vi "Raster_Scan_FSRS.vi"() -> ()   [LabVIEW 2014] (continued)
      n49 = property on="Callibration" class="Bool"("DisabledEnum"=T3."Enabled" ("Disabled")) -> ()  [unwired: 2 in, 2 out]
    }
    frame #2 {
      n50 = while {
        tunnel: w119 -> [w127]
        tunnel: w118 -> [w126]
        tunnel: w117 -> [w125]
        tunnel: w116 -> [w124]
        tunnel: w115 -> [w123]
        tunnel: w114 -> [w122]
        tunnel: w113 -> [w121]
        stop <- "stop" stop-if-true
        n51 = stacked-sequence {
          tunnel: w127 -> [w133 _ _ w229 _ _ _ _]
          tunnel: w126 -> [w132 _ _ w228 _ _ _ _]
          tunnel: w125 -> [w130 _ _ w227 _ _ _ _]
          tunnel: w124 -> [w131 _ _ w226 _ _ _ _]
          tunnel: w123 -> [_ _ _ w223 w358 _ _ _]
          tunnel: w122 -> [w129 _ _ w222 w357 _ _ _]
          tunnel: w121 -> [w128 _ _ w221 w356 _ _ _]
          frame #0 {
            n52 = case shown="True" "winspec" {
              tunnel: w133 -> [_ w142]
              tunnel: w132 -> [_ w141]
              tunnel: w131 -> [_ w139]
              tunnel: w130 -> [_ w138]
              tunnel: w129 -> [_ w136]
              tunnel: w128 -> [_ w135]
              frame False {
              }
              frame True {
                n53 = while {
                  tunnel: w142 -> [w147]
                  tunnel: w141 -> [w148]
                  tunnel: w139 -> [w156]
                  tunnel: w138 -> [w149]
                  stop <- w163 continue-if-true
                  n54 = stacked-sequence {
                    frame #0 {
                      # "This loop continuously updates the graph on the front with the image from the PIXIS"
                      n55 = local read "Camera Handle"() -> (w178:u32)
                      n56 = local read "# Images"() -> (w174:u16)
                      n57 = local read "error out"() -> (w177:errorcluster)
                      n58 = local read "Change to Raman Shift"() -> (w168:bool)
                      n59 = call "DataGrabber.vi"("# Images In"=w174, "Camera Handle"=w178, "error in (no error)"=w177) -> ("# Images Out"=w169:u16, "Camera Handle"=w176:u32, "Data"=w173:dbl[][], "error out"=w175:errorcluster)
                      n60 = case shown="True" w168 {
                        tunnel: [w180 w182] -> w166
                        tunnel: ["Pixel" ("X Scale.Name Label.Text") "Raman Shift (cm-1)" ("X Scale.Name Label.Text")] -> w164
                        frame False {
                          n61 = local read "Result"() -> (w180:dbl[])
                        }
                        frame True {
                          n62 = local read "Result 2"() -> (w182:dbl[])
                        }
                      }
                      n63 = Initialize Array(0.0, u32 1340) -> (w170:dbl[])
                      n64 = call "DataProcessor.vi"("PumpOffBkgd"=w170, "PumpOnBkgd"=w170, "Data"=w173, "# of Images"=w169) -> ("PumpOff"=w167:dbl[])  [unwired: 2 out]
                      n65 = local write "# Images"(w169) -> ()
                      n66 = Build Cluster Array(w166, w167) -> (w165:cluster{dbl, dbl}[])
                      n67 = property on="Spectra" class="XYGraph (strict)"("XScale.NameLbl.Text"=w164) -> ()  [unwired: 2 in, 2 out]
                      n68 = local write "Spectra"(w165) -> ()
                      n69 = local write "Camera Handle"(w176) -> ()
                      n70 = local write "error out"(w175) -> ()
                    }
                    frame #1 {
                      n71 = stacked-sequence {
                        frame #0 {
                          # "Select Cursor 0"
                          n72 = property on="Spectra" class="XYGraph (strict)"("Active Cursor"=0) -> ()  [unwired: 2 in, 2 out]
                        }
                        frame #1 {
                          # "Record the Y position of cursor 0"
                        }
                        frame #2 {
                          # "Select Cursor 1"
                          n73 = property on="Spectra" class="XYGraph (strict)"("Active Cursor"=1) -> ()  [unwired: 2 in, 2 out]
                        }
                        frame #3 {
                          # "Calculate the Gain"
                          n74 = property on="Spectra" class="XYGraph (strict)"() -> ("Cursor.Cursor Position:Cursor Y"=w190:dbl)  [unwired: 2 in, 2 out]
                          n75 = local read "cursor y 2"() -> (w189:dbl)
                          n76 = Subtract(x=w190, y=w189) -> (x-y=w186:dbl)
                          n77 = Absolute Value(x=w186) -> (abs(x)=w188:dbl)
                          n78 = Multiply(x=w188, y=1) -> (x*y=w185:dbl)
                          n79 = local write "Gain"(w185) -> ()
                        }
                      }
                    }
                  }
                  n80 = local read "winspec"() -> (w163:bool)
                  n81 = Boolean To (0,1)(Boolean="PUMP") -> (0, 1=w161:i16)
                  n82 = Multiply(x="Step Size (micro meter)", y=10.0) -> (x*y=w144:dbl)
                  n83 = Add(x=w161, y=i16 1) -> (x+y=w150:i16)
                  n84 = Round To Nearest(number=w144) -> (nearest integer value=w143:dbl)
                  n85 = And(x="MOVE", y=w163) -> (x .and. y?=w157:bool)
                  n86 = call "Pico_move_new.vi"("Motor"=w150, "CmdLib Out"=w147, "DeviceKey Out"=w148, "Start Position"="Start Position", "Boolean 2"="GO", "Relative Steps"=w143, "Boolean"=w157, "error out"=w156, "Device Address Out"=w149) -> ("CmdLib Out"=→"CmdLib Out":refnum<k24>, "DeviceKey Out"=→"DeviceKey Out":string, "Device Address Out"=→"Device Address Out":i32, "error out 2"=→"error out 2":errorcluster)  [unwired: 3 in]
                }
                n87 = call "shutter_new.vi"("error in"=w135, "ShutterID"=310, "Shutter Position"="Shutter Position", "ObjectPtr"=w136) -> ()  [unwired: 1 out]
              }
            }
          }
          frame #1 {
            n88 = case shown="True" "Bkgnd" {
              frame False {
              }
              frame True {
                # "Process the Data"
                # "Get the data!"
                # "Display the Raman Pump on graph on the Front Panel and store data"
                n89 = local read "Camera Handle"() -> (w205:u32)
                n90 = local read "# Images"() -> (w200:u16)
                n91 = local read "error out"() -> (w204:errorcluster)
                n92 = local read "Change to Raman Shift"() -> (w193:bool)
                n93 = call "DataGrabber.vi"("# Images In"=w200, "Camera Handle"=w205, "error in (no error)"=w204) -> ("# Images Out"=w197:u16, "Camera Handle"=w203:u32, "Data"=w201:dbl[][], "error out"=w202:errorcluster)
                n94 = local write "Camera Handle"(w203) -> ()
                n95 = local write "error out"(w202) -> ()
                n96 = local write "# Images"(w197) -> ()
                n97 = case shown="True" w193 {
                  tunnel: [w209 w211] -> w196
                  tunnel: ["Pixel" ("X Scale.Name Label.Text") "Raman Shift (cm-1)" ("X Scale.Name Label.Text")] -> w192
                  frame False {
                    n98 = local read "Result"() -> (w209:dbl[])
                  }
                  frame True {
                    n99 = local read "Result 2"() -> (w211:dbl[])
                  }
                }
                n100 = Initialize Array(0.0) -> (w198:dbl[])  [unwired: 1 in]
                n101 = call "DataProcessor.vi"("PumpOffBkgd"=w198, "PumpOnBkgd"=w198, "Data"=w201, "# of Images"=w197) -> ("PumpOff"=→"Bkgndoff":dbl[], "PumpOn"=→"Bkgndon":dbl[], "Raman"=w195:dbl[])
                n102 = Build Cluster Array(w196, w195) -> (w194:cluster{dbl, dbl}[])
                n103 = property on="Spectra" class="XYGraph (strict)"("XScale.NameLbl.Text"=w192) -> ()  [unwired: 2 in, 2 out]
                n104 = local write "Spectra"(w194) -> ()
              }
            }
          }
          frame #2 {
            n105 = case shown="True" "Callibration" {
              frame False {
              }
              frame True {
                n106 = for {
                  N: 1340 -> [_]
                  tunnel: [w220] -> w219 mode=indexing
                  i -> [w220]
                }
                n107 = call "cal.vi"("array"=w219, "Laser Wavelength"="Laser Wavelength (nm)", "Wave Number"="Shift", "Pixel"="Pixel") -> ("array 2"=→"Result":dbl[], "Result"=→"Result 2":dbl[])  [unwired: 6 in]
              }
            }
          }
          frame #3 {
            n108 = Compound Arithmetic op=OR("Acquire", "Focus") -> (w230:bool)
            n109 = case shown="True" w230 {
              selector: w230 -> [_ w238]
              tunnel: w229 -> [_ w237]
              tunnel: w228 -> [_ w236]
              tunnel: w227 -> [_ w235]
              tunnel: w226 -> [_ w234]
              tunnel: w223 -> [_ w233]
              tunnel: w222 -> [_ w232]
              tunnel: w221 -> [_ w231]
              frame False {
              }
              frame True {
                n110 = while {
                  tunnel: w238 -> [w276]
                  tunnel: w237 -> [w268]
                  tunnel: w236 -> [w267]
                  tunnel: w235 -> [w266]
                  tunnel: w234 -> [w265]
                  tunnel: w233 -> [w244]
                  tunnel: w232 -> [w240]
                  tunnel: w231 -> [w239]
                  stop <- w243 continue-if-true
                  n111 = stacked-sequence {
                    seq-local: [w288 _ _ _] -> [_ w311 _ _]
                    seq-local: [w293 _ _ _] -> [_ w308 _ _]
                    frame #0 {
                      n112 = local read "Camera Handle"() -> (w297:u32)
                      n113 = local read "# Images"() -> (w298:u16)
                      n114 = local read "error out"() -> (w296:errorcluster)
                      n115 = local read "Change to Raman Shift"() -> (w284:bool)
                      n116 = call "DataGrabber.vi"("# Images In"=w298, "Camera Handle"=w297, "error in (no error)"=w296) -> ("# Images Out"=w288:u16, "Camera Handle"=w294:u32, "Data"=w293:dbl[][], "error out"=w295:errorcluster)
                      n117 = case shown="False" w284 {
                        tunnel: [w300 w302] -> w282
                        tunnel: ["Pixel" ("X Scale.Name Label.Text") "Raman Shift (cm-1)" ("X Scale.Name Label.Text")] -> w285
                        frame False {
                          n118 = local read "Result"() -> (w300:dbl[])
                        }
                        frame True {
                          n119 = local read "Result 2"() -> (w302:dbl[])
                        }
                      }
                      n120 = local write "Camera Handle"(w294) -> ()
                      n121 = local write "error out"(w295) -> ()
                      n122 = Initialize Array(0.0, u32 1340) -> (w290:dbl[])
                      n123 = call "DataProcessor.vi"("PumpOffBkgd"=w290, "PumpOnBkgd"=w290, "Data"=w293, "# of Images"=w288) -> ("PumpOff"=w280:dbl[], "PumpOn"=w289:dbl[], "Raman"=w286:dbl[])
                      n124 = local write "# Images"(w288) -> ()
                      n125 = local write "Waveform Graph"(w280) -> ()
                      n126 = property on="Spectra" class="XYGraph (strict)"("XScale.NameLbl.Text"=w285) -> ()  [unwired: 2 in, 2 out]
                      n127 = local write "On"(w289) -> ()
                      n128 = local write "Off"(w280) -> ()
                      n129 = case shown="True" "Flip Spectra" {
                        tunnel: [w303 w304] -> w283
                        tunnel: w286 -> [w303 w305]
                        frame False {
                        }
                        frame True {
                          # "Flip Displayed Spectra"
                          n130 = Reciprocal(x=w305) -> (1/x=w304:dbl[])
                        }
                      }
                      n131 = local write "Raman"(w286) -> ()
                      n132 = Build Cluster Array(w282, w283) -> (w281:cluster{dbl, dbl}[])
                      n133 = local write "Spectra"(w281) -> ()
                    }
                    frame #1 {
                      w315 = 2
                      n134 = Initialize Array(0.0, u32 1340) -> (w319:dbl[])
                      n135 = Initialize Array(0.0, u32 1340) -> (w320:dbl[])
                      n136 = Subtract(x=w311, y=u16 10) -> (x-y=w310:u16)
                      n137 = Divide(x=w311, y=w315) -> (x/y=w316:dbl)
                      n138 = Delete From Array(array=w308, length=10, index (row)=0) -> (array with subset deleted=w307:dbl[][])  [unwired: 1 in, 1 out]
                      n139 = for {
                        N: w310 -> [_]
                        tunnel: w307 -> [w331]
                        shift-right: [w329] -> w318
                        shift-left: w320 -> [w330]
                        shift-right: [w327] -> w317
                        shift-left: w319 -> [w328]
                        tunnel: w315 -> [w326]
                        i -> [w325]
                        n140 = Quotient & Remainder(x=w325, y=w326) -> (x-y*floor(x/y)=w333:i32)  [unwired: 1 out]
                        n141 = Equal To 0?(x=w333) -> (x = 0?=w332:bool)
                        n142 = case shown="True" w332 {
                          tunnel: w331 -> [w338 w345]
                          tunnel: w330 -> [w339 w343]
                          tunnel: [w339 w342] -> w329
                          tunnel: w328 -> [w337 w341]
                          tunnel: [w335 w341] -> w327
                          tunnel: w325 -> [w334 w340]
                          frame False {
                            # "Raman Pump Off\nOdd Images"
                            n143 = Index Array(array=w338, index (row)=w334) -> (element=w336:dbl[])  [unwired: 1 in]
                            n144 = Add(x=w336, y=w337) -> (x+y=w335:dbl[])
                          }
                          frame True {
                            # "Raman pump on\nEven Images"
                            n145 = Index Array(array=w345, index (row)=w340) -> (element=w344:dbl[])  [unwired: 1 in]
                            n146 = Add(x=w344, y=w343) -> (x+y=w342:dbl[])
                          }
                        }
                      }
                      n147 = Divide(x=w318, y=w316) -> (x/y=w313:dbl[])
                      n148 = Divide(x=w317, y=w316) -> (x/y=w314:dbl[])
                      n149 = Divide(x=w313, y=w314) -> ()  [unwired: 1 out]
                    }
                    frame #2 {
                      # "Calculate the Gain based on the two cursors on the graph"
                      n150 = stacked-sequence {
                        frame #0 {
                          # "Select Cursor 0"
                          n151 = property on="Spectra" class="XYGraph (strict)"("Active Cursor"=0) -> ()  [unwired: 2 in, 2 out]
                        }
                        frame #1 {
                          # "Record the Y position of cursor 0"
                          n152 = property on="Spectra" class="XYGraph (strict)"() -> ("Cursor.Cursor Position:Cursor Y"=→"cursor y":dbl)  [unwired: 2 in, 2 out]
                        }
                        frame #2 {
                          # "Select Cursor 1"
                          n153 = property on="Spectra" class="XYGraph (strict)"("Active Cursor"=1) -> ()  [unwired: 2 in, 2 out]
                        }
                        frame #3 {
                          # "Calculate the Gain"
                          n154 = property on="Spectra" class="XYGraph (strict)"() -> ("Cursor.Cursor Position:Cursor Y"=w349:dbl)  [unwired: 2 in, 2 out]
                          n155 = local read "cursor y"() -> (w354:dbl)
                          n156 = Subtract(x=w349, y=w354) -> (x-y=w351:dbl)
                          n157 = Absolute Value(x=w351) -> (abs(x)=w353:dbl)
                          n158 = Multiply(x=w353, y=100) -> (x*y=→"Gain":dbl)
                        }
                      }
                    }
                    frame #3 {
                      n159 = Wait (ms)(milliseconds to wait=50) -> ()  [unwired: 1 out]
                    }
                  }
                  n160 = call <instrlib>:"_subvi_LivePos_Main.vi"("xCommand"="xCommand", "yCommand"="yCommand", "zCommand"="zCommand", "handle"=w244, "commandZ"="commandZ", "commandY"="commandY", "commandX"="commandX") -> ("xRead"=w255:dbl, "yRead"=w254:dbl, "zRead"=w253:dbl, "counter"=w245:u32)  [unwired: 1 in, 8 out]
                  n161 = Equal To 0?(x=w245) -> (x = 0?=w246:bool)
                  n162 = case shown="True" w246 {
                    tunnel: w255 -> [_ w279]
                    tunnel: w254 -> [_ w278]
                    tunnel: w253 -> [_ w277]
                    frame False {
                    }
                    frame True {
                      "xRead" <- w279
                      "yRead" <- w278
                      "zRead" <- w277
                    }
                  }
                  n163 = local read "Shutter Position"() -> (w242:bool)
                  n164 = local read "Focus"() -> (w243:bool)
                  n165 = local read "Step Size (micro meter)"() -> (w259:dbl)
                  n166 = local read "Start Position"() -> (w270:i32)
                  n167 = local read "MOVE"() -> (w272:bool)
                  n168 = local read "PUMP"() -> (w273:bool)
                  n169 = local read "GO"() -> (w264:bool)
                  n170 = Boolean To (0,1)(Boolean=w273) -> (0, 1=w275:i16)
                  n171 = call "shutter_new.vi"("error in"=w239, "ShutterID"=310, "Shutter Position"=w242, "ObjectPtr"=w240) -> ()  [unwired: 1 out]
                  n172 = Add(x=w275, y=i16 1) -> (x+y=w271:i16)
                  n173 = And(x=w272, y=w276) -> (x .and. y?=w269:bool)
                  n174 = Multiply(x=w259, y=10.0) -> (x*y=w257:dbl)
                  n175 = Round To Nearest(number=w257) -> (nearest integer value=w256:dbl)
                  n176 = call "Pico_move_new.vi"("Motor"=w271, "CmdLib Out"=w268, "DeviceKey Out"=w267, "Start Position"=w270, "Boolean 2"=w264, "Relative Steps"=w256, "Boolean"=w269, "error out"=w265, "Device Address Out"=w266) -> ("CmdLib Out"=w263:refnum<k24>, "DeviceKey Out"=w262:string, "Device Address Out"=w261:i32, "error out 2"=w260:errorcluster)  [unwired: 3 in]
                  n177 = local write "CmdLib Out"(w263) -> ()
                  n178 = local write "Device Address Out"(w261) -> ()
                  n179 = local write "error out 2"(w260) -> ()
                  n180 = local write "DeviceKey Out"(w262) -> ()
                }
              }
            }
          }
          frame #4 {
            n181 = case shown="True" "Ruster Scan" {
              tunnel: w358 -> [_ w402]
              tunnel: w357 -> [_ w376]
              tunnel: w356 -> [_ w375]
              frame False {
                (unwired) FALSE ("Pause 2")
              }
              frame True {
                w394 = dbl[][] []
                # "X Ramp Generator"
                # "Y Ramp Generator"
                n182 = local read "Path"() -> (w362:string)
                n183 = Build Array("X Start  (um)", "X End  (um)", "Y Start  (um)", "Y End  (um)") -> (w393:dbl[])
                n184 = Concatenate Strings(w362, "\\" ("string"), "OFF" ("string")) -> (w364:string)
                n185 = Concatenate Strings("Path", "\\" ("string"), "ON" ("string")) -> (w369:string)
                n186 = Array Max & Min(array=w393) -> (max value=w387:dbl)  [unwired: 3 out]
                n187 = String To Path(string=w364) -> (path=w367:path)
                n188 = String To Path(string=w369) -> (path=w373:path)
                n189 = call "RampGenerator.vi"("Number of Positions"="Y Samples", "End  (um)"="Y End  (um)", "Start  (um)"="Y Start  (um)") -> ("Array"=w396:dbl[])  [unwired: 1 in]
                n190 = Greater?(x=w387, y=70.0) -> (0:w377:bool)
                n191 = call "RampGenerator.vi"("Number of Positions"="X Samples", "End  (um)"="X End  (um)", "Start  (um)"="X Start  (um)") -> ("Array"=w397:dbl[])  [unwired: 1 in]
                n192 = case shown="True" w377 {
                  tunnel: [w404 w406] -> w398
                  tunnel: w396 -> [w404 _]
                  tunnel: [w403 w406] -> w399
                  tunnel: w397 -> [w403 _]
                  frame False {
                  }
                  frame True {
                    w406 = dbl[] [] ("Array")
                    n193 = One Button Dialog(message="Values are \nout of Range") -> ()  [unwired: 1 in, 1 out]
                  }
                }
                n194 = Create Folder(path (use dialog)=w367) -> (created path=w363:path)  [unwired: 2 in, 2 out]
                n195 = Create Folder(path (use dialog)=w373) -> (created path=w368:path)  [unwired: 2 in, 2 out]
                n196 = Path To String(path=w363) -> (string=→"OFF":string)
                n197 = Path To String(path=w368) -> (string=→"ON":string)
                n198 = Array Size(array=w396) -> (size(s)=w395:i32)
                n199 = while {
                  tunnel: w398 -> [w448]
                  tunnel: w402 -> [w447]
                  tunnel: w399 -> [w446]
                  tunnel: "X Start  (um)" -> [w445]
                  shift-right: [w440] -> w378
                  shift-left: w394 -> [w424]
                  shift-right: [w442] -> w382
                  shift-left: w394 -> [w423]
                  tunnel: w377 -> [w414]
                  tunnel: w395 -> [w438]
                  tunnel: "X Start  (um)" -> [w437]
                  tunnel: "X End  (um)" -> [w436]
                  tunnel: "Y Start  (um)" -> [w435]
                  tunnel: "Y End  (um)" -> [w434]
                  shift-right: [w429] -> w383
                  shift-left: w394 -> [w425]
                  shift-right: [w427] -> w386
                  shift-left: w394 -> [w426]
                  tunnel: w376 -> [w412]
                  tunnel: w375 -> [w411]
                  i -> [w444]
                  stop <- w413 stop-if-true
                  n200 = Bundle(w426, w425, w424, w423, w414) -> (w422:T5)  [unwired: 1 in]
                  n201 = Unbundle(w422) -> (w421:dbl[][], w418:dbl[][], w420:dbl[][], w419:dbl[][], w410:bool)
                  n202 = stacked-sequence {
                    seq-local: [w450 _] -> [_ w477]
                    tunnel: w448 -> [w454 _]
                    tunnel: w444 -> [w452 w464]
                    tunnel: w447 -> [w453 w478]
                    tunnel: w446 -> [_ w480]
                    tunnel: w445 -> [_ w479]
                    tunnel: [w451 _] -> w408
                    tunnel: [_ w476] -> w417
                    tunnel: [_ w475] -> w416
                    tunnel: [_ w463] -> w433
                    tunnel: w414 -> [_ w474]
                    tunnel: w410 -> [_ w473]
                    tunnel: w438 -> [_ w472]
                    tunnel: w437 -> [_ w471]
                    tunnel: w436 -> [_ w470]
                    tunnel: w435 -> [_ w469]
                    tunnel: w434 -> [_ w468]
                    tunnel: [_ w466] -> w415
                    tunnel: [_ w465] -> w432
                    tunnel: w412 -> [_ w462]
                    tunnel: w411 -> [_ w461]
                    tunnel: [_ w460] -> w407
                    frame #0 {
                      w457 = 2  # Y AXIS
                      # "Step the Y axis"
                      n203 = Array Size(array=w454) -> (size(s)=w449:i32)
                      n204 = Index Array(array=w454, index=w452) -> (element=w455:dbl)
                      n205 = Increment(x=w452) -> (x+1=w456:i32)
                      n206 = Subtract(x=w449, y=w456) -> (x-y=w459:i32)
                      n207 = Equal To 0?(x=w459) -> (x = 0?=w451:bool)
                      n208 = call "WriteReadN.vi"("Handle"=w453, "Axis"=w457, "Delay (ms)"="Y Delay (ms)", "Move to (um)"=w455) -> ("Current Position (um)"=w450:dbl)
                      "Y Position (um)" <- w450
                    }
                    frame #1 {
                      w467 = dbl[] []
                      n209 = while {
                        tunnel: w480 -> [w514]
                        tunnel: w479 -> [w513]
                        tunnel: w478 -> [w511]
                        tunnel: w477 -> [w510]
                        tunnel: w464 -> [w497]
                        shift-right: [w509] -> w476
                        shift-left: w467 -> [w496]
                        shift-right: [w508] -> w475
                        shift-left: w467 -> [w495]
                        tunnel: w474 -> [w507]
                        tunnel: w473 -> [w505]
                        tunnel: w472 -> [w504]
                        tunnel: w471 -> [w503]
                        tunnel: w470 -> [w502]
                        tunnel: w469 -> [w501]
                        tunnel: w468 -> [w500]
                        shift-right: [w499] -> w466
                        shift-left: w467 -> [w494]
                        shift-right: [w498] -> w465
                        shift-left: w467 -> [w490]
                        tunnel: w464 -> [w487]
                        tunnel: [w486] -> w463
                        tunnel: w462 -> [w485]
                        tunnel: w461 -> [w484]
                        tunnel: [w481] -> w460
                        i -> [w512]
                        stop <- w506 stop-if-true
                        n210 = Bundle(w496, w495, w490, w494, w487) -> (w493:cluster{dbl[], dbl[], dbl[], dbl[], i32})  [unwired: 1 in]
                        n211 = Unbundle(w493) -> (w492:dbl[], w491:dbl[], w489:dbl[], w488:dbl[], w486:i32)
                        n212 = stacked-sequence {
                          seq-local: [w532 _] -> [_ w572]
                          tunnel: w514 -> [w537 _]
                          tunnel: w513 -> [_ _]
                          tunnel: w512 -> [w528 _]
                          tunnel: w511 -> [w545 _]
                          tunnel: [w544 _] -> w483
                          tunnel: w510 -> [w543 w573]
                          tunnel: w497 -> [w530 _]
                          tunnel: w492 -> [_ w564]
                          tunnel: [_ w563] -> w509
                          tunnel: [_ w557] -> w508
                          tunnel: w491 -> [_ w566]
                          tunnel: w507 -> [_ _]
                          tunnel: w504 -> [w531 _]
                          tunnel: w503 -> [w520 _]
                          tunnel: w502 -> [w519 _]
                          tunnel: w501 -> [w517 _]
                          tunnel: w500 -> [w518 _]
                          tunnel: w488 -> [_ w561]
                          tunnel: [_ w560] -> w499
                          tunnel: w489 -> [_ w569]
                          tunnel: [_ w567] -> w498
                          tunnel: w485 -> [_ w556]
                          tunnel: w484 -> [_ w555]
                          tunnel: [_ w554] -> w481
                          frame #0 {
                            w546 = 1  # X AXIS
                            # "Step the X axis"
                            n213 = Quotient & Remainder(x=w530, y=2) -> (x-y*floor(x/y)=w541:i32)  [unwired: 1 out]
                            n214 = Array Size(array=w537) -> (size(s)=w529:i32)
                            n215 = Equal?(x=w541, y=0) -> (x = y?=w534:bool)
                            n216 = Multiply(x=w529, y=w530) -> (x*y=w526:i32)
                            n217 = Increment(x=w528) -> (x+1=w527:i32)
                            n218 = Subtract(x=w529, y=1) -> (x-y=w535:i32)
                            n219 = Add(x=w526, y=w527) -> (x+y=w523:i32)
                            n220 = Multiply(x=w531, y=w529) -> (x*y=w522:i32)
                            n221 = Divide(x=w523, y=w522) -> (x/y=w525:dbl)
                            n222 = Subtract(x=w535, y=w528) -> (x-y=w538:i32)
                            n223 = case shown="False" w534 {
                              tunnel: w537 -> [w549 w553]
                              tunnel: w528 -> [_ w552]
                              tunnel: [w550 w551] -> w539
                              tunnel: w538 -> [w548 _]
                              frame False {
                                n224 = Index Array(array=w549, index=w548) -> (element=w550:dbl)
                              }
                              frame True {
                                n225 = Index Array(array=w553, index=w552) -> (element=w551:dbl)
                              }
                            }
                            n226 = Multiply(x=w525, y=100.0) -> (x*y=→"Progress (%)":dbl)
                            n227 = Equal To 0?(x=w538) -> (x = 0?=w544:bool)
                            n228 = Not Equal?(x=w522, y=w523) -> (x != y?=w516:bool)
                            "?" <- w516
                            n229 = call "WriteReadN.vi"("Handle"=w545, "Axis"=w546, "Delay (ms)"="X Deyal (ms)", "Move to (um)"=w539) -> ("Current Position (um)"=w532:dbl)
                            "X Position (um)" <- w532
                            n230 = Not(x=w516) -> (.not. x?=w521:bool)
                            n231 = call "?"("Reset"=w521, "Y Input"=w543, "X Input"=w532) -> ("XY Graph"=→"XY Graph":cluster{"X":dbl[], "Y":dbl[]}[])  [unwired: 7 in, 1 out]
                            n232 = property on="XY Graph" class="XYGraph (strict)"("XScale.Maximum"=w519) -> ()  [unwired: 2 in, 2 out]
                            n233 = property on="XY Graph" class="XYGraph (strict)"("YScale.Minimum"=w517) -> ()  [unwired: 2 in, 2 out]
                            n234 = property on="XY Graph" class="XYGraph (strict)"("YScale.Maximum"=w518) -> ()  [unwired: 2 in, 2 out]
                            n235 = property on="XY Graph" class="XYGraph (strict)"("XScale.Minimum"=w520) -> ()  [unwired: 2 in, 2 out]
                          }
                          frame #1 {
                            w570 = 0.0
                            w571 = 0.0
                            n236 = for {
                              N: "Sets" -> [w593]
                              tunnel: w572 -> [w603]
                              tunnel: w573 -> [w602]
                              shift-right: [w600] -> w562
                              shift-left: w571 -> [w588]
                              shift-right: [w599] -> w565
                              shift-left: w570 -> [w587]
                              shift-right: [w595] -> w568
                              shift-left: w571 -> [w589]
                              shift-right: [w594] -> w558
                              shift-left: w570 -> [w590]
                              tunnel: w556 -> [w580]
                              tunnel: w555 -> [w579]
                              tunnel: [w575] -> w554
                              i -> [w604]
                              n237 = Increment(x=w604) -> (x+1=w581:i32)
                              "Current Set" <- w581
                              n238 = local read item#69() -> (w591:bool)
                              n239 = Bundle(w590, w589, w588, w587) -> (w586:cluster{dbl, dbl, dbl, dbl})  [unwired: 1 in]
                              n240 = Not Equal?(x=w593, y=w581) -> (x != y?=w592:bool)
                              n241 = Not Or(1:w591, 2:w592) -> (0:w577:bool)
                              n242 = Not(x=w577) -> (.not. x?=w576:bool)
                              n243 = stacked-sequence {
                                tunnel: w581 -> [w605 _ _]
                                tunnel: w603 -> [w613 _ _]
                                tunnel: w602 -> [w612 _ _]
                                tunnel: [w611 _ _] -> w601
                                tunnel: [w610 _ _] -> w598
                                tunnel: [w609 _ _] -> w597
                                tunnel: [w608 _ _] -> w596
                                tunnel: w580 -> [w607 _ _]
                                tunnel: w579 -> [w606 _ _]
                                tunnel: [_ _ "STOP Scan"] -> w575
                                frame #0 {
                                n244 = stacked-sequence {
                                seq-local: [_ "# Images" _ _ _ _ _ _] -> [_ _ _ _ _ w698 _ _]
                                seq-local: [_ w622 _ _ _ _ _ _] -> [_ _ w650 _ _ _ w719 _]
                                tunnel: w613 -> [_ _ _ w673 _ _ _ w740]
                                tunnel: w612 -> [_ _ _ w672 _ _ _ w739]
                                tunnel: [_ _ w652 _ _ _ _ _] -> w611
                                tunnel: [_ _ w651 _ _ _ _ _] -> w610
                                tunnel: w605 -> [_ _ _ w674 _ _ _ w741]
                                tunnel: [_ _ _ _ _ _ w718 _] -> w609
                                tunnel: [_ _ _ _ _ _ w717 _] -> w608
                                tunnel: w607 -> [w615 _ _ _ w682 _ _ _]
                                tunnel: w606 -> [w614 _ _ _ w681 _ _ _]
                                frame #0 {
                                n245 = flat-sequence {
                                tunnel: w615 -> [w619]
                                tunnel: w614 -> [w618]
                                frame #0 {
                                n246 = call "shutter_new.vi"("error in"=w618, "ShutterID"=310, "Shutter Position"=TRUE, "ObjectPtr"=w619) -> ()  [unwired: 1 out]
                                }
                                frame #1 {
                                n247 = Wait (ms)(milliseconds to wait=u32 200) -> ()  [unwired: 1 out]
                                }
                                }
                                }
                                frame #1 {
                                n248 = local read "Camera Handle"() -> (w639:u32)
                                n249 = local read "error out"() -> (w638:errorcluster)
                                n250 = call "DataGrabber.vi"("# Images In"="# Images", "Camera Handle"=w639, "error in (no error)"=w638) -> ("# Images Out"=w632:u16, "Camera Handle"=w636:u32, "Data"=w635:dbl[][], "error out"=w637:errorcluster)
                                n251 = case shown="True" "Change to Raman Shift" {
                                tunnel: [w641 w643] -> w622
                                tunnel: ["Pixel" ("X Scale.Name Label.Text") "Raman Shift (cm-1)" ("X Scale.Name Label.Text")] -> w625
                                frame False {
                                n252 = local read "Result"() -> (w641:dbl[])
                                }
                                frame True {
                                n253 = local read "Result 2"() -> (w643:dbl[])
                                }
                                }
                                n254 = local write "Camera Handle"(w636) -> ()
                                n255 = local write "error out"(w637) -> ()
                                n256 = local write "# Images"(w632) -> ()
                                n257 = local read "Bkgndoff"() -> (w633:dbl[])
                                n258 = local read "Bkgndon"() -> (w634:dbl[])
                                n259 = call "DataProcessor.vi"("PumpOffBkgd"=w633, "PumpOnBkgd"=w634, "Data"=w635, "# of Images"=w632) -> ("PumpOff"=w621:dbl[], "PumpOn"=w630:dbl[], "Raman"=w629:dbl[])
                                "Ground" <- w629
                                "On" <- w630
                                "Off" <- w621
                                "Raman" <- w629
                                n260 = local read "Flip Spectra"() -> (w624:bool)
                                n261 = local write "Waveform Graph"(w621) -> ()
                                n262 = property on="Spectra" class="XYGraph (strict)"("XScale.NameLbl.Text"=w625) -> ()  [unwired: 2 in, 2 out]
                                n263 = local write "On"(w630) -> ()
                                n264 = local write "Off"(w621) -> ()
                                n265 = Not(x=w624) -> (.not. x?=w623:bool)
                                n266 = case shown="True" w623 {
                                tunnel: w629 -> [w644 w646]
                                tunnel: [w645 w646] -> w628
                                frame False {
                                n267 = Reciprocal(x=w644) -> (1/x=w645:dbl[])
                                }
                                frame True {
                                }
                                }
                                n268 = Build Cluster Array(w622, w628) -> (→"Spectra":cluster{dbl, dbl}[])
                                }
                                frame #2 {
                                # "Peak fitting and intergation"
                                n269 = local read "Raman"() -> (w653:dbl[])
                                n270 = property on="Spectra" class="XYGraph (strict)"("Active Cursor"=u32 1) -> ("Cursor.Cursor X"=w655:dbl)  [unwired: 2 in, 2 out]
                                n271 = property on="Spectra" class="XYGraph (strict)"("Active Cursor"=u32 0) -> ("Cursor.Cursor X"=w656:dbl)  [unwired: 2 in, 2 out]
                                n272 = call "fit_new.vi"("Filter ?"="Filter?", "parameter bounds"="parameter bounds", "Cursor1 2"=w655, "Cursor1"=w656, "array 2"=w650, "array"=w653, "Enum"="Enum", "Initial Parameters"="Initial Parameters") -> ("Intergrate"=w651:dbl, "Fit"=w652:dbl)  [unwired: 2 in]
                                "FIT" <- w652
                                "AREA" <- w651
                                }
                                frame #3 {
                                # "Here we save spectrum for each special point"
                                n273 = local read "ON"() -> (w667:string)
                                n274 = Format Into String(w674) -> (resulting string=w660:string)  [unwired: 3 in, 1 out]
                                n275 = call "number_to_sring.vi"("Numeric"=w673) -> ("result string"=w665:string)  [unwired: 10 in]
                                n276 = call "number_to_sring.vi"("Numeric"=w672) -> ("result string"=w663:string)  [unwired: 10 in]
                                n277 = Concatenate Strings(w667, "\\", "Filename", "_", "X_" ("string"), w665, "_Y_" ("string"), w663, "_ON" ("string"), "_" ("string"), w660) -> (w671:string)
                                "File_name" <- w671
                                n278 = local read "Ground"() -> (w659:dbl[])
                                n279 = local read "On"() -> (w680:dbl[])
                                n280 = local read "Off"() -> (w679:dbl[])
                                n281 = String To Path(string=w671) -> (path=w677:path)
                                n282 = Build Array(w659, w680, w679) -> (w678:dbl[][])
                                n283 = call-poly <vilib>:"Write To Spreadsheet File.vi"("transpose? (no:F)"=TRUE, "format (%.3f)"="%.7f", "2D data"=w678, "file path (dialog if empty)"=w677) -> ()  [unwired: 4 in, 1 out]
                                }
                                frame #4 {
                                n284 = flat-sequence {
                                tunnel: w682 -> [w686]
                                tunnel: w681 -> [w685]
                                frame #0 {
                                n285 = call "shutter_new.vi"("error in"=w685, "ShutterID"=310, "Shutter Position"=FALSE, "ObjectPtr"=w686) -> ()  [unwired: 1 out]
                                }
                                frame #1 {
                                n286 = Wait (ms)(milliseconds to wait=u32 200) -> ()  [unwired: 1 out]
                                }
                                }
                                }
                                frame #5 {
                                n287 = local read "Camera Handle"() -> (w706:u32)
                                n288 = local read "error out"() -> (w705:errorcluster)
                                n289 = local read "Change to Raman Shift"() -> (w694:bool)
                                n290 = call "DataGrabber.vi"("# Images In"=w698, "Camera Handle"=w706, "error in (no error)"=w705) -> ("# Images Out"=w699:u16, "Camera Handle"=w703:u32, "Data"=w702:dbl[][], "error out"=w704:errorcluster)
                                n291 = local write "Camera Handle"(w703) -> ()
                                n292 = local write "error out"(w704) -> ()
                                n293 = local write "# Images"(w699) -> ()
                                n294 = local read "Bkgndoff"() -> (w700:dbl[])
                                n295 = local read "Bkgndon"() -> (w701:dbl[])
                                n296 = case shown="False" w694 {
                                tunnel: [w708 w710] -> w693
                                tunnel: ["Pixel" ("X Scale.Name Label.Text") "Raman Shift (cm-1)" ("X Scale.Name Label.Text")] -> w695
                                frame False {
                                n297 = local read "Result"() -> (w708:dbl[])
                                }
                                frame True {
                                n298 = local read "Result 2"() -> (w710:dbl[])
                                }
                                }
                                n299 = call "DataProcessor.vi"("PumpOffBkgd"=w700, "PumpOnBkgd"=w701, "Data"=w702, "# of Images"=w699) -> ("PumpOff"=w688:dbl[], "PumpOn"=w697:dbl[], "Raman"=w696:dbl[])
                                n300 = local read "Flip Spectra"() -> (w690:bool)
                                n301 = local write "Waveform Graph"(w688) -> ()
                                n302 = Not(x=w690) -> (.not. x?=w689:bool)
                                n303 = local write "On"(w697) -> ()
                                n304 = local write "Off"(w688) -> ()
                                n305 = case shown="True" w689 {
                                tunnel: w696 -> [w712 w713]
                                tunnel: [w711 w713] -> w692
                                frame False {
                                n306 = Reciprocal(x=w712) -> (1/x=w711:dbl[])
                                }
                                frame True {
                                }
                                }
                                n307 = property on="Spectra" class="XYGraph (strict)"("XScale.NameLbl.Text"=w695) -> ()  [unwired: 2 in, 2 out]
                                n308 = local write "Ground"(w696) -> ()
                                n309 = local write "Raman"(w696) -> ()
                                n310 = Build Cluster Array(w693, w692) -> (w691:cluster{dbl, dbl}[])
                                n311 = local write "Off"(w688) -> ()
                                n312 = local write "Spectra"(w691) -> ()
                                n313 = local write "On"(w697) -> ()
                                }
                                frame #6 {
                                # "Peak fitting and intergation"
                                n314 = local read "Raman"() -> (w720:dbl[])
                                n315 = local read "Initial Parameters"() -> (w721:T2)
                                n316 = local read "Enum"() -> (w716:enum16{"Lorantzian", "fano", "gaussian"})
                                n317 = property on="Spectra" class="XYGraph (strict)"("Active Cursor"=u32 0) -> ("Cursor.Cursor X"=w723:dbl)  [unwired: 2 in, 2 out]
                                n318 = property on="Spectra" class="XYGraph (strict)"("Active Cursor"=u32 1) -> ("Cursor.Cursor X"=w722:dbl)  [unwired: 2 in, 2 out]
                                n319 = local read "Filter?"() -> (w714:bool)
                                n320 = local read "parameter bounds"() -> (w715:T1)
                                n321 = call "fit_new.vi"("Filter ?"=w714, "parameter bounds"=w715, "Cursor1 2"=w722, "Cursor1"=w723, "array 2"=w719, "array"=w720, "Enum"=w716, "Initial Parameters"=w721) -> ("Intergrate"=w717:dbl, "Fit"=w718:dbl)  [unwired: 2 in]
                                n322 = local write "AREA"(w717) -> ()
                                n323 = local write "FIT"(w718) -> ()
                                }
                                frame #7 {
                                # "Here we save spectrum for each special point"
                                n324 = local read "Filename"() -> (w736:string)
                                n325 = Format Into String(w741) -> (resulting string=w727:string)  [unwired: 3 in, 1 out]
                                n326 = call "number_to_sring.vi"("Numeric"=w740) -> ("result string"=w732:string)  [unwired: 10 in]
                                n327 = local read "OFF"() -> (w734:string)
                                n328 = call "number_to_sring.vi"("Numeric"=w739) -> ("result string"=w730:string)  [unwired: 10 in]
                                n329 = Concatenate Strings(w734, "\\", w736, "_", "X_" ("string"), w732, "_Y_" ("string"), w730, "_OFF" ("string"), "_" ("string"), w727) -> (w738:string)
                                n330 = local read "Ground"() -> (w726:dbl[])
                                n331 = local read "Off"() -> (w747:dbl[])
                                n332 = local read "Off"() -> (w746:dbl[])
                                n333 = String To Path(string=w738) -> (path=w744:path)
                                n334 = local write "File_name"(w738) -> ()
                                n335 = Build Array(w726, w747, w746) -> (w745:dbl[][])
                                n336 = call-poly <vilib>:"Write To Spreadsheet File.vi"("transpose? (no:F)"=TRUE, "format (%.3f)"="%.7f", "2D data"=w745, "file path (dialog if empty)"=w744) -> ()  [unwired: 4 in, 1 out]
                                }
                                }
                                }
                                frame #1 {
                                n337 = stacked-sequence {
                                frame #0 {
                                n338 = property on="Spectra" class="XYGraph (strict)"("Active Cursor"=0) -> ()  [unwired: 2 in, 2 out]
                                }
                                frame #1 {
                                n339 = property on="Spectra" class="XYGraph (strict)"() -> ("Cursor.Cursor Position:Cursor Y"=w749:dbl)  [unwired: 2 in, 2 out]
                                n340 = local write "cursor y"(w749) -> ()
                                }
                                frame #2 {
                                n341 = property on="Spectra" class="XYGraph (strict)"("Active Cursor"=1) -> ()  [unwired: 2 in, 2 out]
                                }
                                frame #3 {
                                n342 = property on="Spectra" class="XYGraph (strict)"() -> ("Cursor.Cursor Position:Cursor Y"=w751:dbl)  [unwired: 2 in, 2 out]
                                n343 = local read "cursor y"() -> (w752:dbl)
                                n344 = Subtract(x=w751, y=w752) -> (x-y=w754:dbl)
                                n345 = Absolute Value(x=w754) -> (abs(x)=w756:dbl)
                                n346 = Multiply(x=w756, y=100) -> (x*y=w753:dbl)
                                n347 = local write "Gain"(w753) -> ()
                                }
                                }
                                }
                                frame #2 {
                                n348 = while {
                                stop <- "Pause" continue-if-true
                                }
                                }
                              }
                              n349 = Not(x=w575) -> (.not. x?=w574:bool)
                              n350 = And(x=w576, y=w574) -> (x .and. y?=→"Scanig":bool)
                              n351 = Unbundle(w586) -> (w585:dbl, w584:dbl, w583:dbl, w582:dbl)
                              n352 = Add(x=w598, y=w582) -> (x+y=w599:dbl)
                              n353 = Add(x=w596, y=w585) -> (x+y=w594:dbl)
                              n354 = Add(x=w601, y=w583) -> (x+y=w600:dbl)
                              n355 = Add(x=w597, y=w584) -> (x+y=w595:dbl)
                            }
                            n356 = call "array.vi"("x"=w558, "y"="Sets", "array"=w561) -> ("appended array"=w560:dbl[])  [unwired: 6 in]
                            n357 = call "array.vi"("x"=w562, "y"="Sets", "array"=w564) -> ("appended array"=w563:dbl[])  [unwired: 6 in]
                            n358 = call "array.vi"("x"=w565, "y"="Sets", "array"=w566) -> ("appended array"=w557:dbl[])  [unwired: 6 in]
                            n359 = call "array.vi"("x"=w568, "y"="Sets", "array"=w569) -> ("appended array"=w567:dbl[])  [unwired: 6 in]
                          }
                        }
                        n360 = Or(x=w483, y=w481) -> (x .or. y?=w482:bool)
                        n361 = Or(x=w505, y=w482) -> (x .or. y?=w506:bool)
                      }
                    }
                  }
                  n362 = Or(x=w408, y=w407) -> (x .or. y?=w409:bool)
                  n363 = Or(x=w410, y=w409) -> (x .or. y?=w413:bool)
                  n364 = call "rotate.vi"("Array in"=w432, "i"=w433) -> ("Array out"=w430:dbl[])  [unwired: 9 in]
                  n365 = call "rotate.vi"("Array in"=w415, "i"=w433) -> ("Array out"=w431:dbl[])  [unwired: 9 in]
                  n366 = call "rotate.vi"("Array in"=w416, "i"=w433) -> ("Array out"=w443:dbl[])  [unwired: 9 in]
                  n367 = call "rotate.vi"("Array in"=w417, "i"=w433) -> ("Array out"=w441:dbl[])  [unwired: 9 in]
                  n368 = Build Array (concatenate)(w430, w421) -> (w427:dbl[][])
                  n369 = Transpose 2D Array(2D array=w427) -> (transposed array=→"DCP OFF":dbl[][])
                  n370 = Build Array (concatenate)(w431, w418) -> (w429:dbl[][])
                  n371 = Build Array (concatenate)(w441, w420) -> (w440:dbl[][])
                  n372 = Transpose 2D Array(2D array=w440) -> (transposed array=→"DCP ON":dbl[][])
                  n373 = Build Array (concatenate)(w443, w419) -> (w442:dbl[][])
                }
                n374 = local read "Filename"() -> (w374:string)
                n375 = local read "Path"() -> (w379:string)
                n376 = call "save_file.vi"("string 3"="_area_ON" ("string"), "string 2"=w374, "string"=w379, "2D data"=w382) -> ()  [unwired: 8 in]
                n377 = call "save_file.vi"("string 3"="_fit_ON" ("string"), "string 2"=w374, "string"=w379, "2D data"=w378) -> ()  [unwired: 8 in]
                n378 = call "save_file.vi"("string 3"="_area_OFF" ("string"), "string 2"=w374, "string"=w379, "2D data"=w383) -> ()  [unwired: 8 in]
                n379 = call "save_file.vi"("string 3"="_fit_OFF" ("string"), "string 2"=w374, "string"=w379, "2D data"=w386) -> ()  [unwired: 8 in]
              }
            }
          }
          frame #5 {
            n380 = case shown="True" "takefsrs" {
              frame False {
              }
              frame True {
                n381 = for {
                  N: "Sets 2" -> [w761]
                  i -> [w762]
                  # "This \"For Loop\" loops over the desired number of sets the user would like to take"
                  n382 = stacked-sequence {
                    tunnel: w762 -> [w768 w770]
                    tunnel: w761 -> [_ w771]
                    frame #0 {
                      # "Here we figure out the frequency with which we need to take grounds to take the proper number"
                      # "Need to increment by 1"
                      # "Scramble the timepoints before beginning a new set"
                      n383 = local read "Timepoints"() -> (w766:dbl[])
                      n384 = Increment(x=w768) -> (x+1=→"Current Set 2":i32)
                      n385 = local read "#Ground"() -> (w765:u32)
                      n386 = Array Size(array=w766) -> (size(s)=w764:i32)
                      n387 = call "randomize.vi"("Input array"=w766) -> ("Output array"=w769:dbl[])
                      n388 = Quotient & Remainder(x=w764, y=w765) -> (floor(x/y)=→"GndNum":u32)  [unwired: 1 out]
                      n389 = local write "Timepoints"(w769) -> ()
                    }
                    frame #1 {
